vi "Generate Tx Data.vi"(8 "error in (no error)":errorcluster, 11 "OPC UA in":refnum<class "OPC UA.lvclass">) -> (0 "error out":errorcluster, 2 "Tx Data":variant, 3 "OPC UA out":refnum<class "OPC UA.lvclass">)   [LabVIEW 2021, in "OPC UA.lvclass"]
uses:
  OPC UA.lvclass
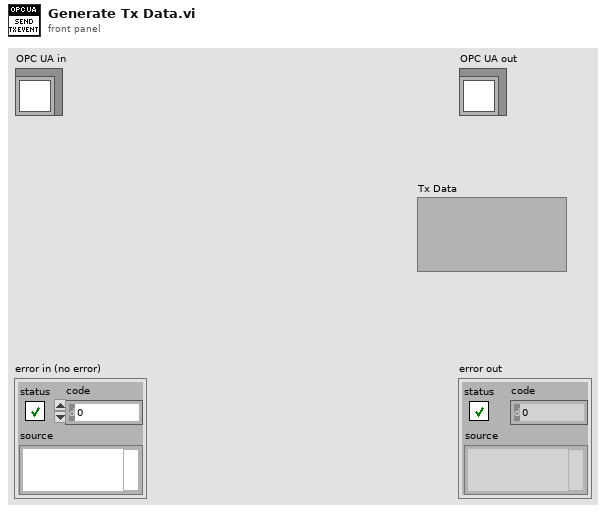
[diagram p1: front panel]
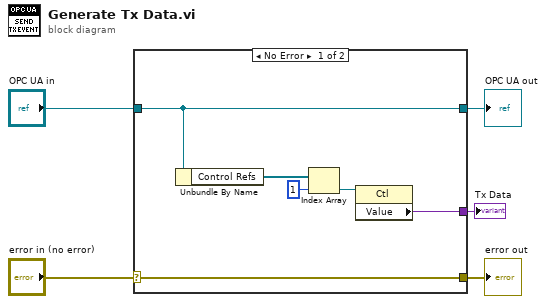
[diagram p0: block diagram]
diagram:
  n1 = case shown="No Error" "error in (no error)" {
    selector: "error in (no error)" -> [w11 w13]
    tunnel: [w11 w13] -> w4
    tunnel: [w8 w12] -> w2
    tunnel: "OPC UA in" -> [w8 w12]
    tunnel: [w6 _] -> w1
    frame No Error {
      n2 = Unbundle By Name(w8) -> ("Control Refs"=w7:refnum<vi>[])
      n3 = Index Array(array=w7, index=1) -> (element=w10:refnum<vi>)
      n4 = property class="Ctl"(reference=w10) -> ("Value"=w6:variant)  [unwired: 1 in, 2 out]
    }
    frame Error {
    }
  }
  "error out" <- w4
  "OPC UA out" <- w2
  "Tx Data" <- w1
